vi "Fold Matrix.vi"(9 "Index":i32, 10 "Coordenate":string, 11 "Dots Matrix":bool[][](array[boolean])) -> (3 "Result":bool[][](array[boolean]))   [LabVIEW 2019, in "Day 13.lvlib"]
uses:
  Day 13.lvlib
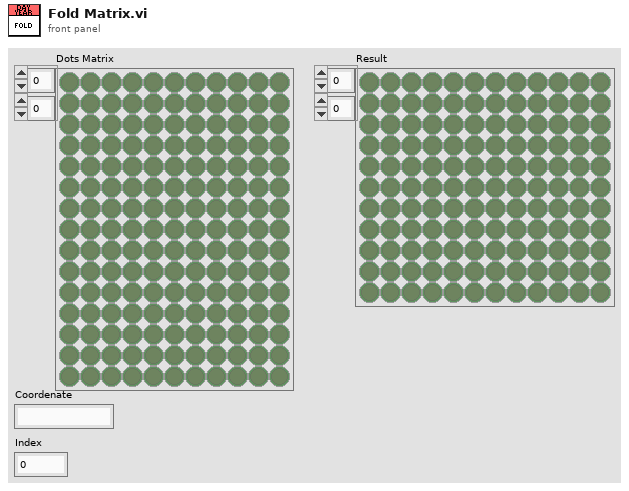
[diagram p1: front panel]
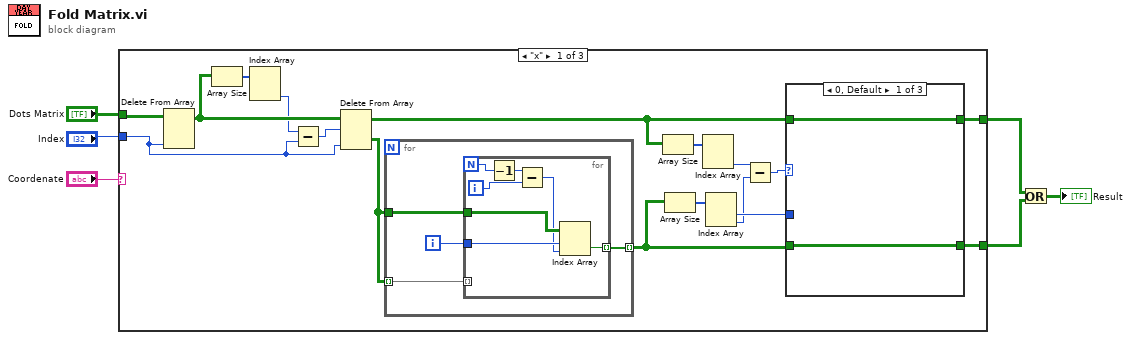
[diagram p0: block diagram]
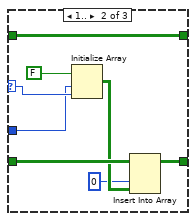
[diagram p2: hidden frame]
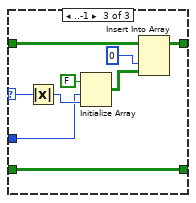
[diagram p3: hidden frame]
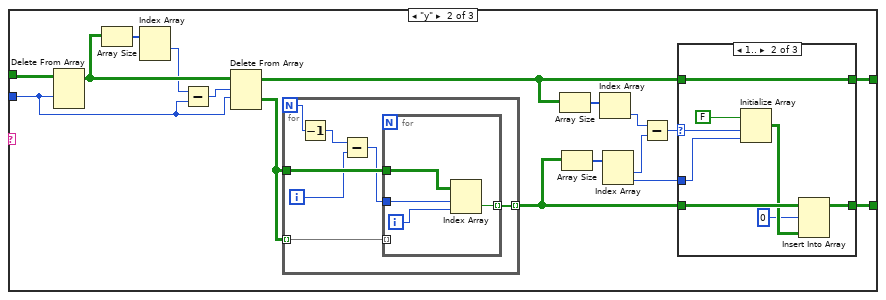
[diagram p4: hidden frame]
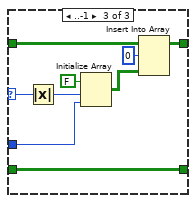
[diagram p6: hidden frame]
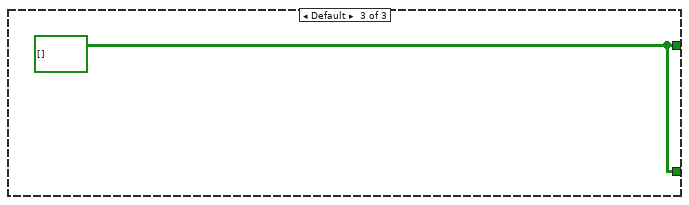
[diagram p7: hidden frame]
diagram:
  n1 = case shown="\"x\"" "Coordenate" {
    tunnel: "Dots Matrix" -> [w23 w70 _]
    tunnel: "Index" -> [w18 w65 _]
    tunnel: [w16 w56 w101] -> w2
    tunnel: [w15 w55 w101] -> w1
    frame "x" {
      n2 = Delete From Array(array=w23, index (col)=w18) -> (array with subset deleted=w22:bool[][])  [unwired: 2 in, 1 out]
      n3 = Array Size(array=w22) -> (size(s)=w21:i32[])
      n4 = Index Array(array=w21) -> (element #2=w19:i32)  [unwired: 2 in, 1 out]
      n5 = Subtract(x=w19, y=w18) -> (x-y=w20:i32)
      n6 = Delete From Array(array=w22, length=w20, index (col)=w18) -> (deleted portion=w17:bool[][], array with subset deleted=w12:bool[][])  [unwired: 1 in]
      n7 = for {
        tunnel: w17 -> [w46]
        tunnel: w17 -> [w44] mode=indexing
        tunnel: [w43] -> w11 mode=indexing
        i -> [w45]
        n8 = for {
          N -> [w48]
          tunnel: w46 -> [w53]
          tunnel: w45 -> [w52]
          tunnel: w44 -> [_] mode=indexing
          tunnel: [w50] -> w43 mode=indexing
          i -> [w51]
          n9 = Decrement(x=w48) -> (x-1=w47:i32)
          n10 = Subtract(x=w47, y=w51) -> (x-y=w49:i32)
          n11 = Index Array(array=w53, index (row)=w52, index (col)=w49) -> (element=w50:bool)
        }
      }
      n12 = Array Size(array=w12) -> (size(s)=w14:i32[])
      n13 = Array Size(array=w11) -> (size(s)=w13:i32[])
      n14 = Index Array(array=w14) -> (element #2=w10:i32)  [unwired: 2 in, 1 out]
      n15 = Index Array(array=w13) -> (element #1=w9:i32, element #2=w8:i32)  [unwired: 2 in]
      n16 = Subtract(x=w10, y=w8) -> (x-y=w7:i32)
      n17 = case shown="0, Default" w7 {
        selector: w7 -> [_ w28 w40]
        tunnel: w12 -> [w25 w29 w39]
        tunnel: w11 -> [w24 w33 w37]
        tunnel: [w25 w29 w38] -> w16
        tunnel: [w24 w30 w37] -> w15
        tunnel: w9 -> [_ w27 w35]
        frame 0, Default {
        }
        frame 1.. {
          n18 = Initialize Array(FALSE, w27, w28) -> (w31:bool[][])
          n19 = Insert Into Array(array=w33, index (col)=0 ("index (row)"), new element=w31) -> (w30:bool[][])  [unwired: 1 in]
        }
        frame ..-1 {
          n20 = Absolute Value(x=w40) -> (abs(x)=w36:i32)
          n21 = Initialize Array(FALSE, w35, w36) -> (w41:bool[][])
          n22 = Insert Into Array(array=w39, index (col)=0 ("index (row)"), new element=w41) -> (w38:bool[][])  [unwired: 1 in]
        }
      }
    }
    frame "y" {
      n23 = Delete From Array(array=w70, index (row)=w65) -> (array with subset deleted=w69:bool[][])  [unwired: 2 in, 1 out]
      n24 = Array Size(array=w69) -> (size(s)=w68:i32[])
      n25 = Index Array(array=w68) -> (element #1=w66:i32)  [unwired: 2 in, 1 out]
      n26 = Subtract(x=w66, y=w65) -> (x-y=w67:i32)
      n27 = Delete From Array(array=w69, length=w67, index (row)=w65) -> (deleted portion=w64:bool[][], array with subset deleted=w58:bool[][])  [unwired: 1 in]
      n28 = for {
        N -> [w91]
        tunnel: w64 -> [w96]
        tunnel: w64 -> [w95] mode=indexing
        tunnel: [w94] -> w57 mode=indexing
        i -> [w93]
        n29 = Decrement(x=w91) -> (x-1=w90:i32)
        n30 = Subtract(x=w90, y=w93) -> (x-y=w92:i32)
        n31 = for {
          tunnel: w96 -> [w100]
          tunnel: w92 -> [w99]
          tunnel: w95 -> [_] mode=indexing
          tunnel: [w98] -> w94 mode=indexing
          i -> [w97]
          n32 = Index Array(array=w100, index (row)=w99, index (col)=w97) -> (element=w98:bool)
        }
      }
      n33 = Array Size(array=w58) -> (size(s)=w63:i32[])
      n34 = Array Size(array=w57) -> (size(s)=w62:i32[])
      n35 = Index Array(array=w63) -> (element=w61:i32)  [unwired: 1 in]
      n36 = Index Array(array=w62) -> (element #1=w60:i32, element #2=w54:i32)  [unwired: 2 in]
      n37 = Subtract(x=w61, y=w60) -> (x-y=w59:i32)
      n38 = case shown="1.." w59 {
        selector: w59 -> [_ w78 w86]
        tunnel: w58 -> [w72 w73 w83]
        tunnel: w57 -> [w71 w80 w81]
        tunnel: [w72 w73 w82] -> w56
        tunnel: [w71 w74 w81] -> w55
        tunnel: w54 -> [_ w77 w84]
        frame 0, Default {
        }
        frame 1.. {
          n39 = Initialize Array(FALSE, w78, w77) -> (w76:bool[][])
          n40 = Insert Into Array(array=w80, index (row)=0, new element=w76) -> (w74:bool[][])  [unwired: 1 in]
        }
        frame ..-1 {
          n41 = Absolute Value(x=w86) -> (abs(x)=w85:i32)
          n42 = Initialize Array(FALSE, w85, w84) -> (w88:bool[][])
          n43 = Insert Into Array(array=w83, index (row)=0, new element=w88) -> (w82:bool[][])  [unwired: 1 in]
        }
      }
    }
    frame Default {
      w101 = bool[][] [] ("Dots Matrix")
    }
  }
  n44 = Or(x=w2, y=w1) -> (x .or. y?=→"Result":bool[][])
